vi "Idle Pattern and Sounds.vi"() -> ()   [LabVIEW 2026]
uses:
  <vilib>/rvi/Emulation/niFpgaGetClockAttributes.vi
  <vilib>/rvi/Emulation/niFpgaSctlEmulationGetInTimedLoop.vi
  <vilib>/rvi/Emulation/niFpgaEmulationReportErrorSimple.vi
  <instrlib>/_niInstr/Basic Elements/v1/FPGA/Private/Count Up U16.vi
  <vilib>/rvi/eio/common/nirviEmuTemplateMethod_errors.vi
  <vilib>/rvi/Emulation/niFpgaCriticalErrorInLSC.vi
  <vilib>/eio/EIONode/EIONode.xnode
  <instrlib>/_niInstr/Basic Elements/v1/FPGA/niInstr Basic Elements v1 FPGA.lvlib
  <vilib>/rvi/DataTransferAndStorage/Container/XNode/niFpgaContainer.xnode
  <vilib>/rvi/interface/RandomDataEmulation/nirviRandomDataFpgaReadWriteTemplate.vi
panel:
  in  "End Audio Loop":bool
  in  "Turn On Audio":bool
  out "Timed Out?":bool
  in  "Count(Ticks)":u32=907 caption="Audio Loop Time"
  in  "x":u16[](array[numeric])=[0, 0, 0, 0, 0, 0, 0, 0, 0, 0, 0, 0, 0, 0, 0, 0, 0, 0, 0, 0, 0, 0, 0, 0, 0, 0, 0, 0, 0, 0, 0, 0, 0, 0, 0, 0, 0, 0, 0, 0, 0, 0, 0, 0, 0]
  out "Numeric":i32
  in  "Period":u16=100
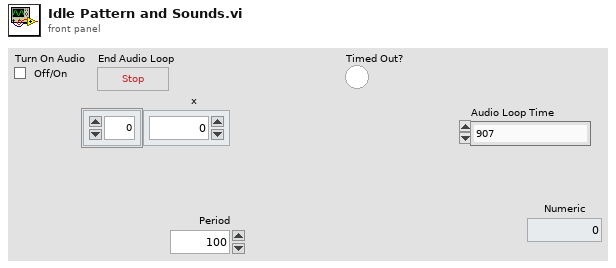
[diagram p1: front panel]
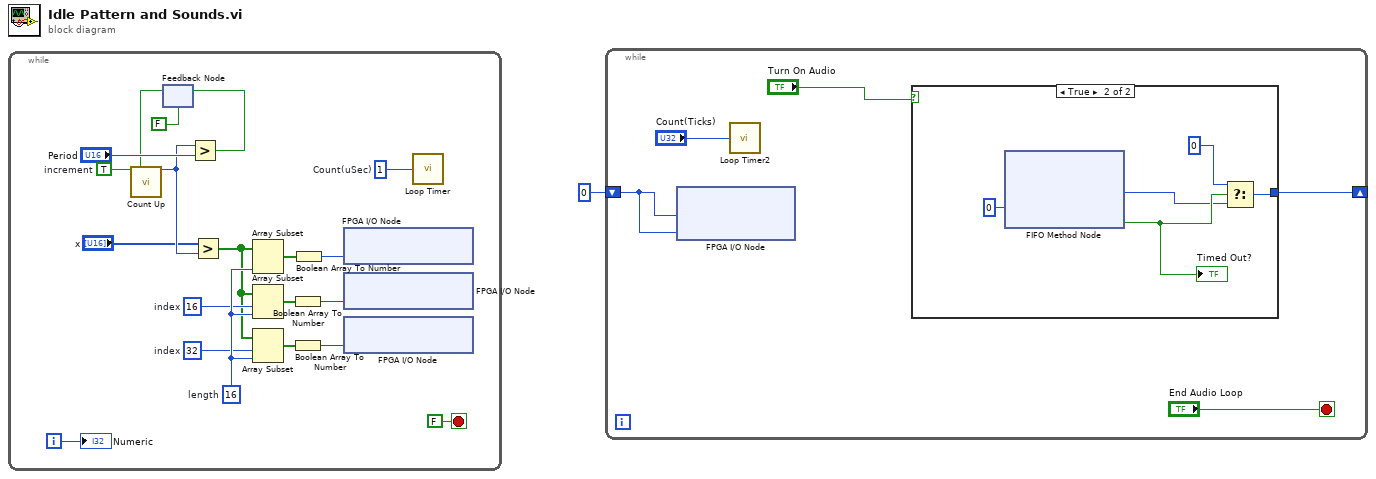
[diagram p0: block diagram]
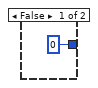
[diagram p2: hidden frame]
diagram:
  n1 = while {
    i -> [w18]
    stop <- FALSE stop-if-true
    w6 = 32  # index
    w7 = 16  # index
    w8 = 16  # length
    w16 = u16 1  # Count(uSec)
    w20 = TRUE  # increment
    n2 = feedback #1(FALSE) -> (w15:bool)
    n3 = call-poly <instrlib>:"Count Up.vi"("increment"=w20, "reset"=w15) -> ("count out"=w13:u16)  [unwired: 13 in]
    n4 = Greater?(x=w13, y="Period") -> (0:w17:bool)
    n5 = feedback-in #1(w17) -> ()
    n6 = Greater?(x="x", y=w13) -> (0:w4:bool[])
    n7 = Array Subset(array=w4, length=w8) -> (w2:bool[])  [unwired: 1 in]
    n8 = Array Subset(array=w4, index=w7, length=w8) -> (w3:bool[])
    n9 = Array Subset(array=w4, index=w6, length=w8) -> (w5:bool[])
    n10 = Boolean Array To Number(Boolean array=w3) -> (number=w10:u16)
    n11 = Boolean Array To Number(Boolean array=w5) -> (number=w9:u16)
    n12 = Boolean Array To Number(Boolean array=w2) -> (number=w11:u16)
    n13 = xnode "FPGA I/O Node"("Bank-01/DO15:0"=w11) -> ()  [unwired: 1 in, 1 out]
    n14 = xnode "FPGA I/O Node"("Bank-02/DO15:0"=w10) -> ()  [unwired: 1 in, 1 out]
    n15 = xnode "FPGA I/O Node"("Bank-03/DO15:0"=w9) -> ()  [unwired: 1 in, 1 out]
    n16 = call "Loop Timer"("Count(uSec)"=w16) -> ()  [unwired: 1 out]
    "Numeric" <- w18
  }
  n17 = while {
    shift-right: [w25] -> _
    shift-left: i16 0 ("SteroOut/AO0") -> [w26]
    stop <- "End Audio Loop" stop-if-true
    n18 = xnode "FPGA I/O Node"("SteroOut/AO0"=w26, "SteroOut/AO1"=w26) -> ()  [unwired: 2 in, 2 out]
    n19 = call "Loop Timer2"("Count(Ticks)"="Count(Ticks)") -> ()  [unwired: 1 out]
    n20 = case shown="True" "Turn On Audio" {
      tunnel: [i16 0 ("Element") w29] -> w25
      frame False {
      }
      frame True {
        n21 = xnode ("FIFO Method Node")("Timeout"=0) -> ("Element"=w30:i16, "Timed Out?"=w31:bool)  [unwired: 1 in, 1 out]
        "Timed Out?" <- w31
        n22 = Select(t=i16 0, s=w31, f=w30) -> (s? t:f=w29:i16)
      }
    }
  }
